vi "Set Working Directory.vi"(8 "error in (no error)":errorcluster, 10 "New Path (/usb1/)":string="/usb1/", 11 "VISA resource name":refnum<visa-resource-name>) -> (0 "error out":errorcluster, 2 "Current Working Directory":string, 3 "VISA resource name out":refnum<visa-resource-name>)   [LabVIEW 2015, in "Keithley 2600 Series.lvlib"]
doc: "Sets the current working directory."
uses:
  Keithley 2600 Series.lvlib
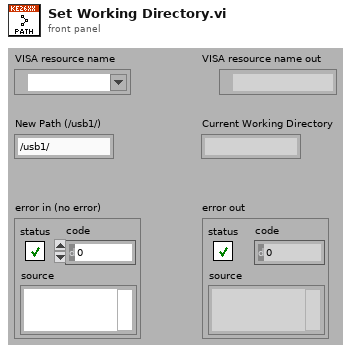
[diagram p1: front panel]
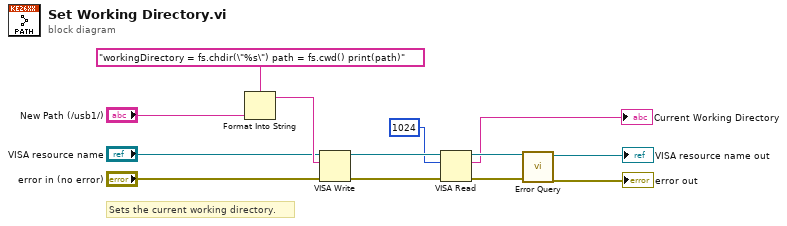
[diagram p0: block diagram]
diagram:
  # "Sets the current working directory."
  n1 = Format Into String(format string="workingDirectory = fs.chdir(\"%s\") path = fs.cwd() print(path)", "New Path (/usb1/)") -> (resulting string=w11:string)  [unwired: 2 in, 1 out]
  n2 = VISA Write(VISA resource name="VISA resource name", write buffer=w11, error in (no error)="error in (no error)") -> (VISA resource name out=w6:refnum<visa-resource-name>, error out=w5:errorcluster)  [unwired: 1 out]
  n3 = VISA Read(VISA resource name=w6, byte count=u32 1024, error in (no error)=w5) -> (VISA resource name out=w4:refnum<visa-resource-name>, read buffer=→"Current Working Directory":string, error out=w3:errorcluster)  [unwired: 1 out]
  n4 = call "Error Query.vi"("error in (no error)"=w3, "VISA resource name"=w4) -> ("error out"=→"error out":errorcluster, "VISA resource name out"=→"VISA resource name out":refnum<visa-resource-name>)  [unwired: 6 in, 2 out]
